vi "ni579x IQ Impairment Correction.vi"(7 "scope":string="rx", 8 "Error In":errorcluster, 10 "frequency [Hz]":dbl=200000000.0 format="%#_6p", 11 "characterization data":T2 {"Frequencies [Hz]" format="%#_6p"}) -> (0 "Error Out":errorcluster, 1 "uncorrected carrier gain":dbl, 2 "correction gain":dbl, 3 "IQ impairment correction out":T1)   [LabVIEW 2015]
uses:
  <instrlib>/ni579x/Config/v1/Shared/Types/ni579x Characterization Data.ctl
  <instrlib>/ni579x/Config/v1/Shared/Types/ni579x IQ Imbalance.ctl
  <instrlib>/ni579x/Config/v1/Shared/Types/ni579x Gain to Attenuation Mapping.ctl
  <instrlib>/_niInstr/DSP/v1/Shared/Public/IQ Impairments.ctl
  <instrlib>/_niInstr/DSP/v1/Shared/niInstr DSP v1 Shared.lvlib
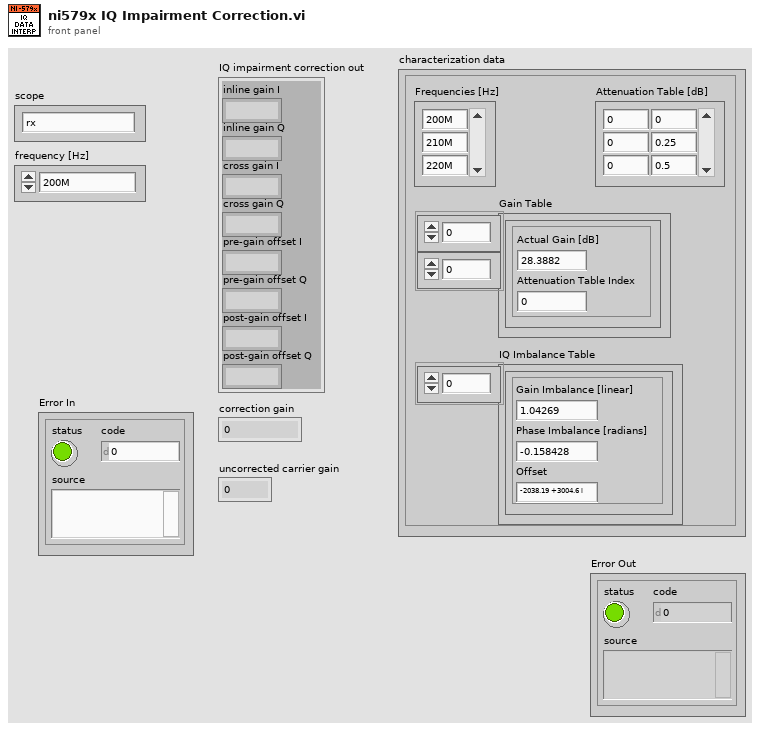
[diagram p1: front panel]
types:
  T1 = typedef "niInstr DSP v1 Shared.lvlib/IQ Impairments.ctl" = cluster{"inline gain I":fxp<+/-,18,1>, "inline gain Q":fxp<+/-,18,1>, "cross gain I":fxp<+/-,18,1>, "cross gain Q":fxp<+/-,18,1>, "pre-gain offset I":fxp<+/-,18,1>, "pre-gain offset Q":fxp<+/-,18,1>, "post-gain offset I":fxp<+/-,18,1>, "post-gain offset Q":fxp<+/-,18,1>}
  T2 = typedef "ni579x Characterization Data.ctl" = cluster{"Attenuation Table [dB]":dbl[][], "Frequencies [Hz]":dbl[], "IQ Imbalance Table":T3[], "Gain Table":T4[][]}
  T3 = typedef "ni579x IQ Imbalance.ctl" = cluster{"Gain Imbalance [linear]":dbl, "Phase Imbalance [radians]":dbl, "Offset":cdb}
  T4 = typedef "ni579x Gain to Attenuation Mapping.ctl" = cluster{"Actual Gain [dB]":dbl, "Attenuation Table Index":i32}
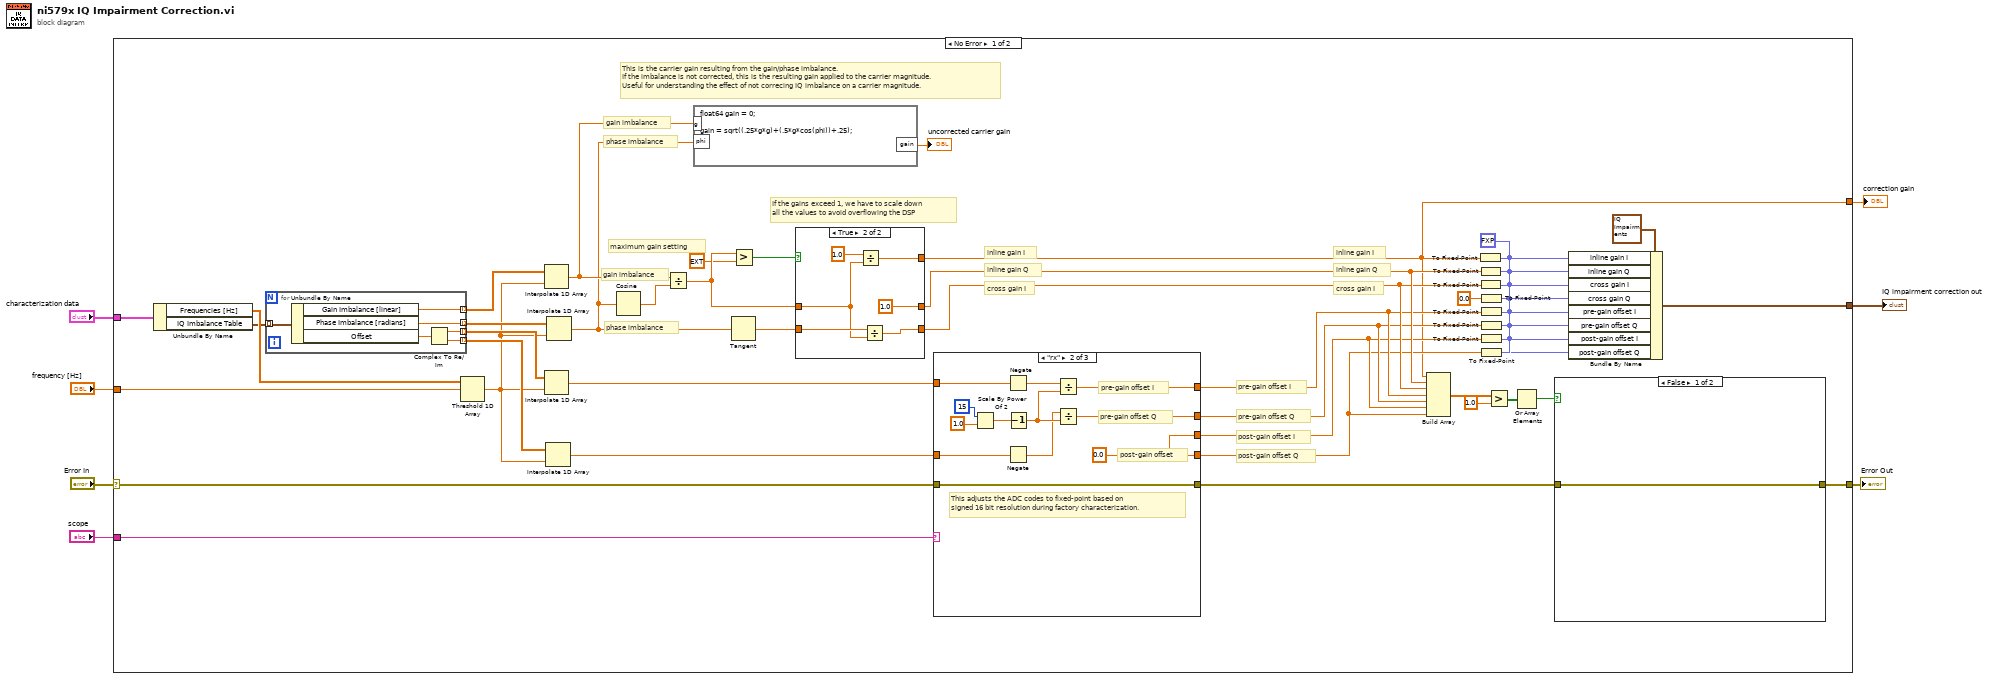
[diagram p0: block diagram]
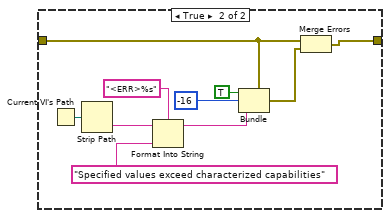
[diagram p2: hidden frame]
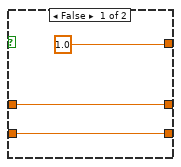
[diagram p3: hidden frame]
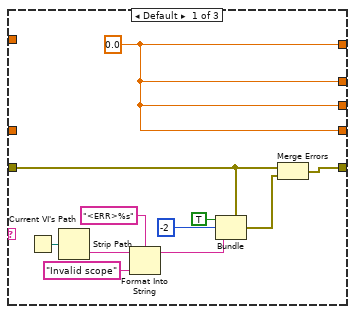
[diagram p4: hidden frame]
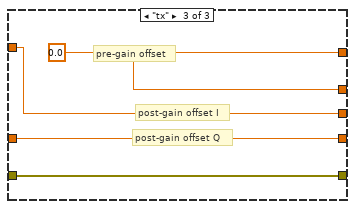
[diagram p5: hidden frame]
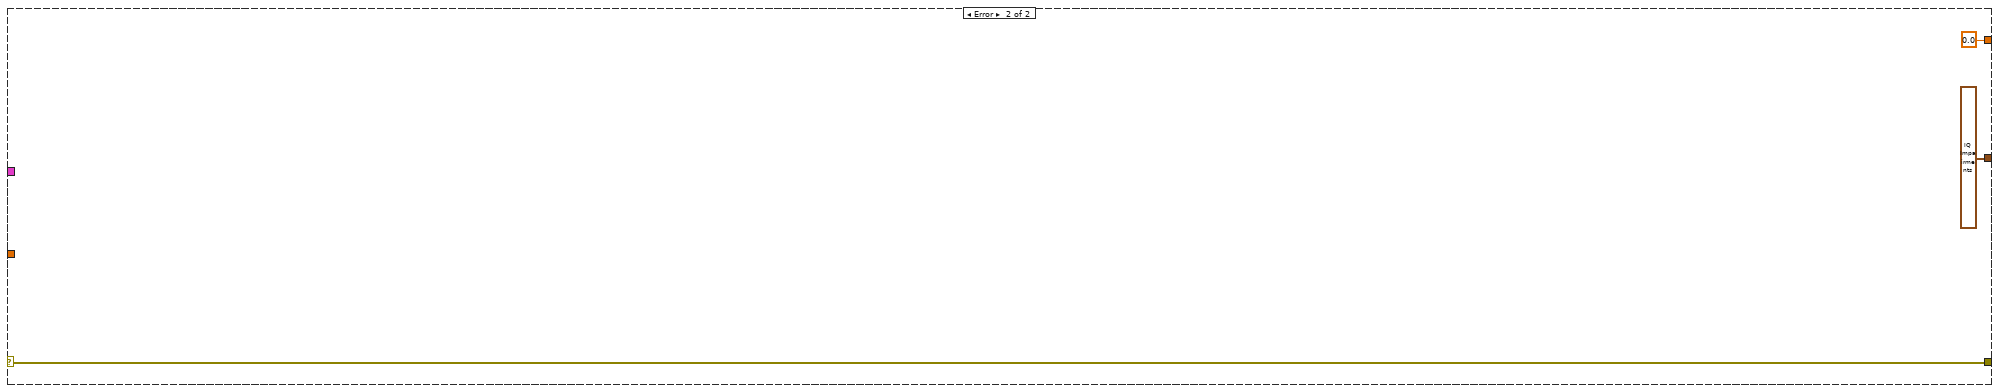
[diagram p6: hidden frame]
diagram:
  n1 = case shown="No Error" "Error In" {
    selector: "Error In" -> [w52 w109]
    tunnel: [w14 w109] -> w4
    tunnel: "frequency [Hz]" -> [w44 _]
    tunnel: "characterization data" -> [w46 _]
    tunnel: "scope" -> [w53 _]
    tunnel: [w12 0.0 ("number")] -> w2
    tunnel: [w13 T1 {"inline gain I"=0.9999923706054688, "inline gain Q"=0.9999923706054688, "cross gain I"=0.0, "cross gain Q"=0.0, "pre-gain offset I"=0.0, "pre-gain offset Q"=0.0, "post-gain offset I"=0.0, "post-gain offset Q"=0.0} ("IQ impairment out")] -> w1
    frame No Error {
      w35 = fxp<+/-,18,1> 0.0 ("cross gain I")
      # "This is the carrier gain resulting from the gain/phase imbalance.\nIf the imbalance is not corrected, this is the resulting gain applied to the carrier magnitude.\nUseful for understanding the effect of not correcing IQ imbalance on a carrier magnitude."
      # "phase imbalance"
      # "gain imbalance"
      # "If the gains exceed 1, we have to scale down\nall the values to avoid overflowing the DSP"
      # "phase imbalance"
      # "gain imbalance"
      # "post-gain offset Q"
      # "post-gain offset I"
      # "pre-gain offset Q"
      # "pre-gain offset I"
      # "cross gain I"
      # "inline gain Q"
      # "inline gain I"
      # "cross gain I"
      # "inline gain Q"
      # "inline gain I"
      # "maximum gain setting"
      n2 = Unbundle By Name(w46) -> ("Frequencies [Hz]"=w50:dbl[], "IQ Imbalance Table"=w47:T3[])
      n3 = for {
        tunnel: w47 -> [w79] mode=indexing
        tunnel: [w78] -> w49 mode=indexing
        tunnel: [w77] -> w48 mode=indexing
        tunnel: [w75] -> w51 mode=indexing
        tunnel: [w74] -> w45 mode=indexing
        n4 = Unbundle By Name(w79) -> ("Gain Imbalance [linear]"=w78:dbl, "Phase Imbalance [radians]"=w77:dbl, "Offset"=w76:cdb)
        n5 = Complex To Re/Im(x + iy=w76) -> (x=w75:dbl, y=w74:dbl)
      }
      n6 = Threshold 1D Array(2:w44, 3:w50) -> (0:w11:dbl)  [unwired: 1 in]
      n7 = Interpolate 1D Array(1:w11, 2:w49) -> (0:w10:dbl)
      n8 = Interpolate 1D Array(1:w11, 2:w51) -> (0:w41:dbl)
      n9 = Interpolate 1D Array(1:w11, 2:w45) -> (0:w42:dbl)
      n10 = Interpolate 1D Array(1:w11, 2:w48) -> (0:w9:dbl)
      n11 = Cosine(x=w9) -> (cos(x)=w43:dbl)
      n12 = Divide(x=w10, y=w43) -> (x/y=w39:dbl)
      n13 = formula code="float64 gain = 0;\n\ngain = sqrt((.25*g*g)+(.5*g*cos(phi))+.25);"("g"=w10, "phi"=w9) -> ("gain"=→"uncorrected carrier gain":dbl)
      n14 = Tangent(1:w9) -> (0:w38:dbl)
      n15 = Greater?(x=w39, y=ext 1.0 ("number")) -> (0:w40:bool)
      n16 = case shown="True" w40 {
        tunnel: w39 -> [w66 w71]
        tunnel: w38 -> [w65 w73]
        tunnel: [1.0 ("number") w70] -> w12
        tunnel: [w66 1.0] -> w25
        tunnel: [w65 w68] -> w24
        frame False {
        }
        frame True {
          n17 = Divide(x=1.0 ("number"), y=w71) -> (x/y=w70:dbl)
          n18 = Divide(x=w73, y=w71) -> (x/y=w68:dbl)
        }
      }
      n19 = case shown="\"rx\"" w53 {
        tunnel: w41 -> [_ w94 w105]
        tunnel: [w82 w96 w106] -> w15
        tunnel: w52 -> [w81 w96 w106]
        tunnel: w42 -> [_ w95 w104]
        tunnel: [w80 w93 w103] -> w23
        tunnel: [w80 w92 w103] -> w22
        tunnel: [w80 w91 w105] -> w21
        tunnel: [w80 w91 w104] -> w20
        frame Default {
          w80 = 0.0
          n20 = Current VI's Path() -> (path=w84:path)
          n21 = Strip Path(path=w84) -> (name=w85:string)  [unwired: 1 out]
          n22 = Format Into String(format string="<ERR>%s", initial string=w85, "Invalid scope" ("input 1")) -> (resulting string=w86:string)  [unwired: 1 in, 1 out]
          n23 = Bundle(cluster=w81, "status"=TRUE, "code"=-2, "source"=w86) -> (w87:errorcluster)
          n24 = Merge Errors(w81, w87) -> (w82:errorcluster)
        }
        frame "rx" {
          w91 = 0.0
          # "post-gain offset"
          # "pre-gain offset Q"
          # "pre-gain offset I"
          # "This adjusts the ADC codes to fixed-point based on \nsigned 16 bit resolution during factory characterization."
          n25 = Scale By Power Of 2(n=15, x=1.0) -> (x*2^n=w100:dbl)
          n26 = Negate(x=w94) -> (-x=w98:dbl)
          n27 = Negate(x=w95) -> (-x=w97:dbl)
          n28 = Decrement(x=w100) -> (x-1=w101:dbl)
          n29 = Divide(x=w98, y=w101) -> (x/y=w93:dbl)
          n30 = Divide(x=w97, y=w101) -> (x/y=w92:dbl)
        }
        frame "tx" {
          w103 = 0.0
          # "post-gain offset Q"
          # "post-gain offset I"
          # "pre-gain offset"
        }
      }
      n31 = Build Array(w12, w25, w24, w23, w22, w21, w20) -> (w19:dbl[])
      n32 = To Fixed-Point(fixed-point type=w35, number=w12) -> (fixed-point=w33:fxp<+/-,18,1>)
      n33 = To Fixed-Point(fixed-point type=w35, number=w25) -> (fixed-point=w32:fxp<+/-,18,1>)
      n34 = To Fixed-Point(fixed-point type=w35, number=w24) -> (fixed-point=w31:fxp<+/-,18,1>)
      n35 = To Fixed-Point(fixed-point type=w35, number=0.0) -> (fixed-point=w30:fxp<+/-,18,1>)
      n36 = To Fixed-Point(fixed-point type=w35, number=w23) -> (fixed-point=w29:fxp<+/-,18,1>)
      n37 = To Fixed-Point(fixed-point type=w35, number=w22) -> (fixed-point=w28:fxp<+/-,18,1>)
      n38 = To Fixed-Point(fixed-point type=w35, number=w21) -> (fixed-point=w27:fxp<+/-,18,1>)
      n39 = To Fixed-Point(fixed-point type=w35, number=w20) -> (fixed-point=w26:fxp<+/-,18,1>)
      n40 = Greater?(x=w19, y=1.0) -> (0:w17:bool[])
      n41 = Or Array Elements(Boolean array=w17) -> (logical OR=w16:bool)
      n42 = case shown="False" w16 {
        tunnel: w15 -> [w54 w56]
        tunnel: [w54 w55] -> w14
        frame False {
        }
        frame True {
          n43 = Current VI's Path() -> (path=w58:path)
          n44 = Strip Path(path=w58) -> (name=w59:string)  [unwired: 1 out]
          n45 = Format Into String(format string="<ERR>%s", initial string=w59, "Specified values exceed characterized capabilities" ("input 1")) -> (resulting string=w60:string)  [unwired: 1 in, 1 out]
          n46 = Bundle(cluster=w56, "status"=TRUE, "code"=-16, "source"=w60) -> (w61:errorcluster)
          n47 = Merge Errors(w56, w61) -> (w55:errorcluster)
        }
      }
      n48 = Bundle By Name(cluster=T1 {"inline gain I"=0.9999923706054688, "inline gain Q"=0.9999923706054688, "cross gain I"=0.0, "cross gain Q"=0.0, "pre-gain offset I"=0.9999923706054688, "pre-gain offset Q"=0.9999923706054688, "post-gain offset I"=0.0, "post-gain offset Q"=0.0} ("IQ impairment out"), "inline gain I"=w33, "inline gain Q"=w32, "cross gain I"=w31, "cross gain Q"=w30, "pre-gain offset I"=w29, "pre-gain offset Q"=w28, "post-gain offset I"=w27, "post-gain offset Q"=w26) -> (w13:T1)
    }
    frame Error {
    }
  }
  "IQ impairment correction out" <- w1
  "Error Out" <- w4
  "correction gain" <- w2
